vi "Do.vi"(8 "error in (no error)":errorcluster, 10 "Actor in":refnum<class "Actor.lvclass">, 11 "Stop Nested Actors Msg":refnum<class "Stop Nested Actors Msg.lvclass">) -> (0 "error out":errorcluster, 2 "Actor out":refnum<class "Actor.lvclass">)   [LabVIEW 2020, in "Actor with Nesteds.lvlib" / "Stop Nested Actors Msg.lvclass"]
doc: "<p>(<strong>Filename</strong>: <span class=\"dnl\">Actor Framework.lvlib:Message.lvclass:Do.vi</span>)</p>\n<p>Defines what a message does when it is received by an actor. Generally, a message instructs an actor to invoke one of its methods. By default, this method does nothing. A child class must override it to define behavior.</p>"
uses:
  Stop Nested Actors Msg.lvclass
  Core/ActorFramework/Actor/Actor.lvclass
  Actor with Nesteds/Actor with Nesteds.lvclass
  C:/Users/J63553/Projects/_LabVIEW Community/actor-framework/Core/ActorFramework/Actor/Actor.lvclass
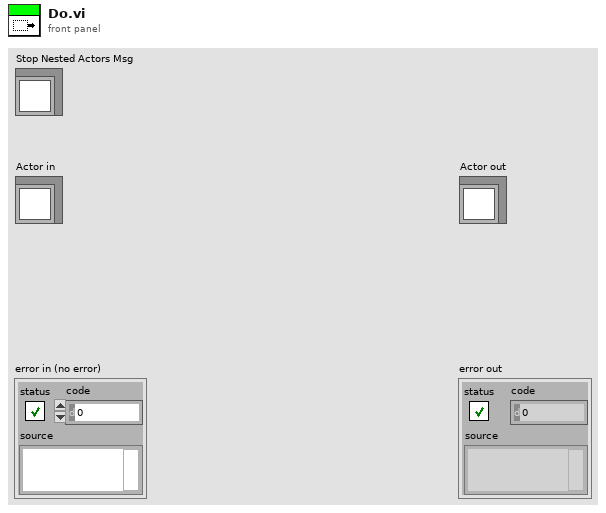
[diagram p1: front panel]
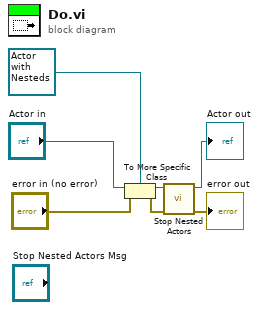
[diagram p0: block diagram]
diagram:
  n1 = To More Specific Class(target class=refnum<class "Actor with Nesteds.lvclass"> refnum ("Actor with Nesteds.lvlib:Actor with Nesteds.lvclass"), reference="Actor in", error in="error in (no error)") -> (specific class reference=w4:refnum<class "Actor with Nesteds.lvclass">, error out=w2:errorcluster)
  n2 = call "Stop Nested Actors.vi"("error in (no error)"=w2, "Actor with Nesteds in"=w4) -> ("error out"=→"error out":errorcluster, "Actor with Nesteds out"=→"Actor out":refnum<class "Actor with Nesteds.lvclass">)  [unwired: 8 in]
